vi "A-Lockin_Vsg.vi"(8 "error in (no error)":errorcluster, 9 "Channels: AO":T1={"AO amp (V)"=[0.0002, 0.0, 0.0, 0.0, 0.0, 0.0, 0.0, 0.0], "AO DC (V)"=[0.00025, 0.0, 0.0, 0.0, 0.0, 0.0, 0.0, 0.0], "AO f (Hz)"=[13.0, 13.0, 13.0, 13.0, 13.0, 13.0, 13.0, 13.0], "AO phi (deg)"=[0.0, 0.0, 0.0, 0.0, 0.0, 0.0, 0.0, 0.0], "function"=[enum."Sine Wave", enum."Sine Wave", enum."Sine Wave", enum."Sine Wave", enum."Sine Wave", enum."Sine Wave", enum."Sine Wave", enum."Sine Wave"]} {"AO f (Hz)" min=0.001 max=10000.0; "AO DC (V)" format="%#_6p"; "AO amp (V)" format="%#_6p"}, 10 "Comments":string="SA03036H\nsweep Vsg:-150m to 700m, 500u steps\nB 7T to -7T\nVbg =-3.9V\nT: 50mK\n\nlockin\n\nI+/-: 4/28 200uV ac+ 250u dc bias, 13Hz\nV1+/-: 3/27\nV2+/- 2/6\nV3+/V3-: 7/8\nVsg: 1\nVbg :26\n\ntc 300ms order 2", 11 "ITX folder":string="4L4Lockinfieldsweep") -> (0 "error out":errorcluster)   [LabVIEW 2016, in "Transport.lvclass"]
uses:
  Transport.lvclass
  <userlib>/LevyLab/Lockin-Multichannel/Typedefs/AO-cluster.ctl
  <userlib>/LevyLab/Lockin-Multichannel/Typedefs/AO_Amp-array.ctl
  <userlib>/LevyLab/Lockin-Multichannel/Typedefs/AO_DC-array.ctl
  <userlib>/LevyLab/Lockin-Multichannel/Typedefs/AO_f-array.ctl
  <userlib>/LevyLab/Lockin-Multichannel/Typedefs/AO_phi-array.ctl
  <userlib>/LevyLab/Lockin-Multichannel/Typedefs/Function-array.ctl
  <userlib>/LevyLab/Lockin-Multichannel/Typedefs/Function-enum.ctl
  SMOs/SweepControl/SweepControl.lvclass
  subVI/ITX_Global.vi
  <userlib>/LevyLab/Levylab Instruments/Instrument.lvclass
  <userlib>/LevyLab/LV to ITX/LVtoITX.lvclass
panel:
  in  "Tab Control":enum32{"lockin/SG Control", "Data"}(tab)
  in  "SweepControl.lvclass":refnum<class "SweepControl.lvclass">
  in  "Vmax (end)":dbl=0.7 format="%#_3p"
  in  "Vmin (start)":dbl=-0.15 format="%#_3p"
  in  "dV":dbl=0.0005 format="%#_3p"
  out "T (mK)":dbl
  in  "wait after setting Vsg (ms)":u32
  in  "Initial wait (ms)":u32=10000
  in  "side gate channel":i32=1
  in  "Physical Channel":tag="Dev2/ao0" caption="Back Gate Channel"
  in  "Sweep":enum16{"Vsg", "Vbg"}(ring)
  in  "cycles (1,2,...)":i32=1 min=1 step=1
  in  "phase":dbl
  out "ramp rate":dbl=0.2 format="%#_13g"
  out "Field":dbl=0.5 format="%#_13g"
  in  "function (ramp)":enum16{"Ramp", "Triangle", "Sine"}(ring)
  in  "set \"Vsg\" to initial value?":bool
  out "time (ms)":u32=76
  out "G 4T":cluster{"Y":dbl[], "Y":dbl[]}[](graph)
  out "Lockins":cluster{"Y":dbl[], "Y":dbl[]}[](graph)
  out "Lockins 2":cluster{"Y":dbl[], "Y":dbl[]}[](graph)
  # "0"
  # "1"
  # "2"
  # "3"
  # "4"
  # "5"
  # "6"
  # "7"
  # "dynamically name the traces"
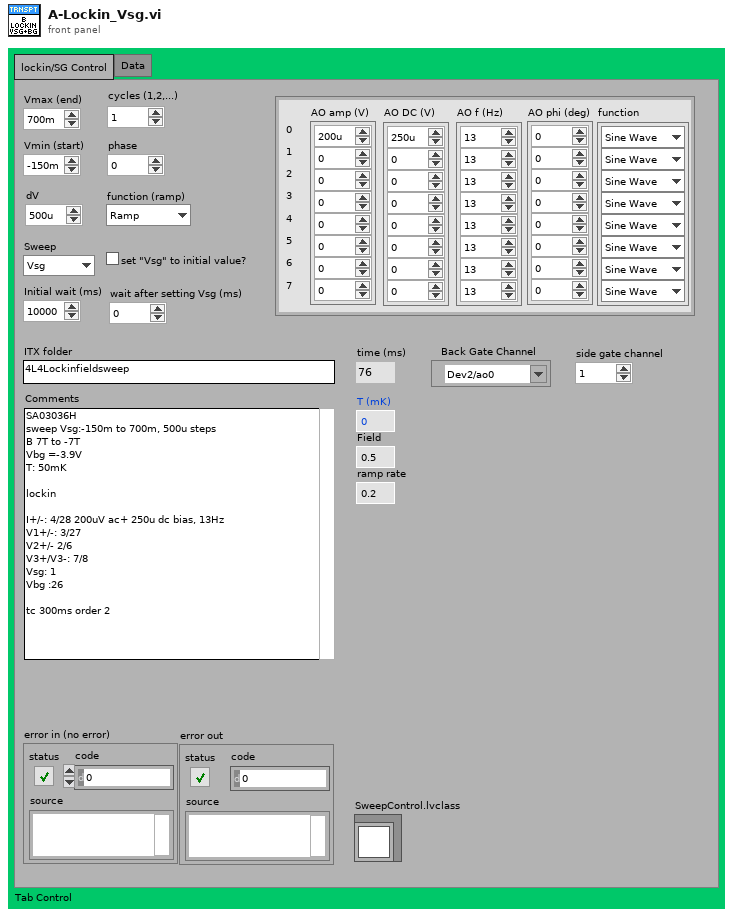
[diagram p1: front panel]
types:
  T1 = typedef "AO-cluster.ctl" = cluster{"AO amp (V)":T2, "AO DC (V)":T3, "AO f (Hz)":T4, "AO phi (deg)":T5, "function":T6}
  T2 = typedef "AO_Amp-array.ctl" = dbl[]
  T3 = typedef "AO_DC-array.ctl" = dbl[]
  T4 = typedef "AO_f-array.ctl" = dbl[]
  T5 = typedef "AO_phi-array.ctl" = dbl[]
  T6 = typedef "Function-array.ctl" = T7[]
  T7 = typedef "Function-enum.ctl" = enum16{"Sine Wave", "Triangle Wave", "Square Wave", "Sawtooth Wave"}
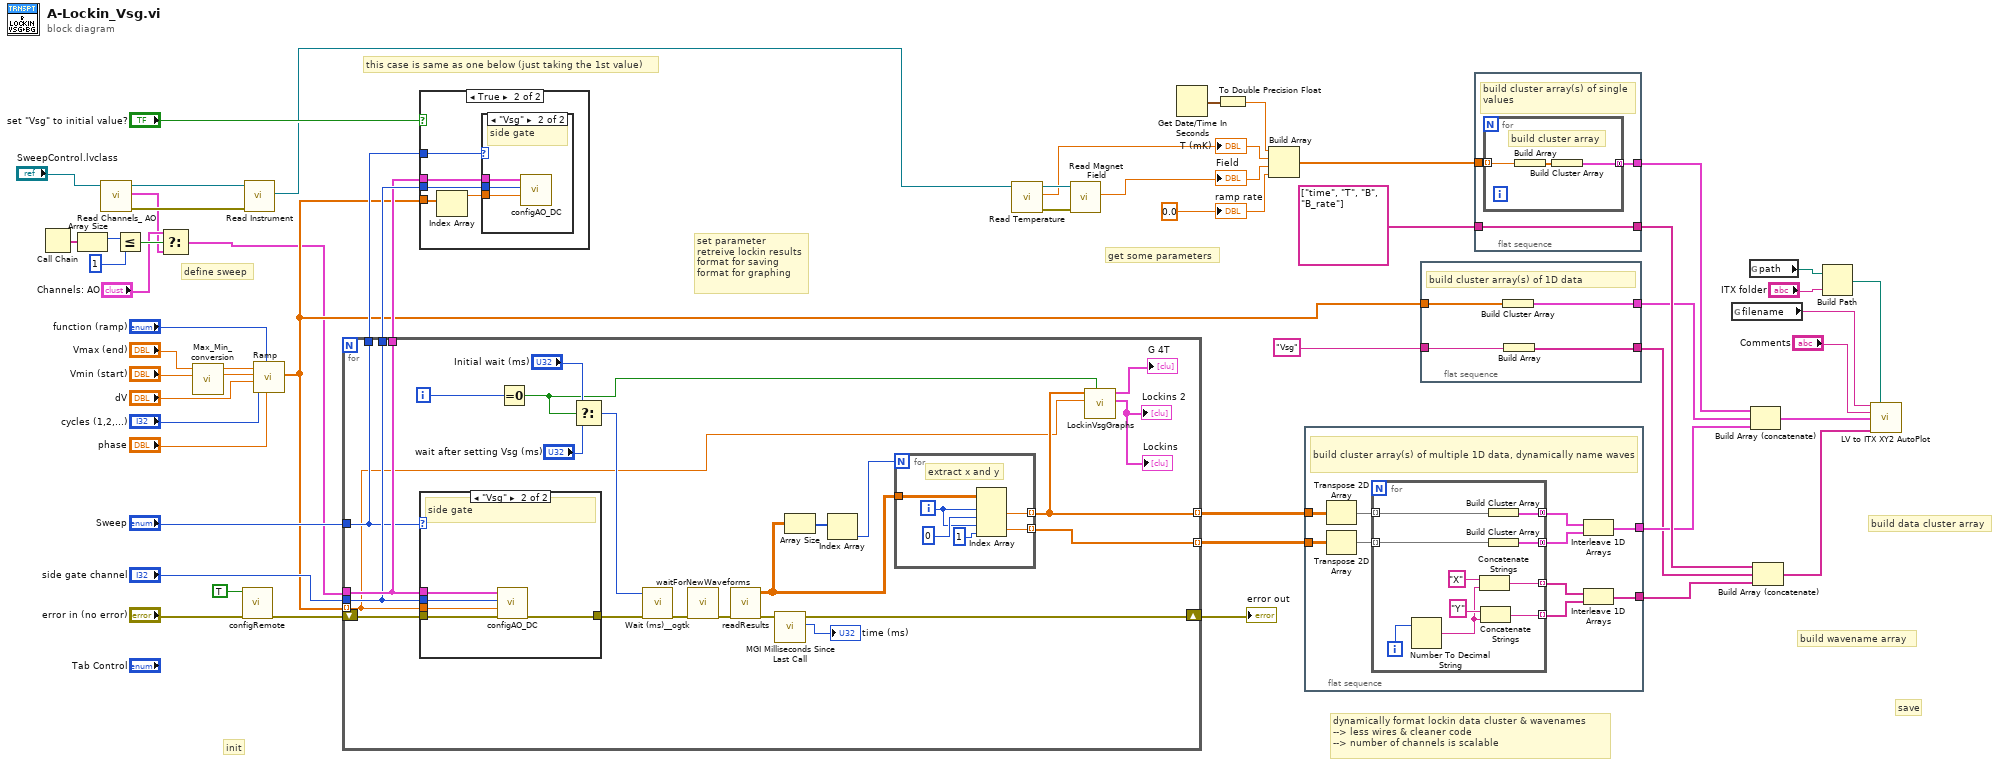
[diagram p0: block diagram]
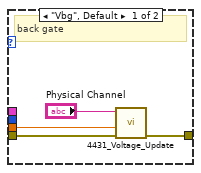
[diagram p2: hidden frame]
diagram:
  w19 = 0.0
  # "define sweep"
  # "get some parameters"
  # "set parameter\nretreive lockin results\nformat for saving\nformat for graphing"
  # "save"
  # "this case is same as one below (just taking the 1st value)"
  # "init"
  # "build data cluster array"
  # "build wavename array"
  # "dynamically format lockin data cluster & wavenames\n--> less wires & cleaner code\n--> number of channels is scalable"
  n1 = Call Chain() -> (call chain=w7:string[])
  n2 = Array Size(array=w7) -> (size(s)=w6:i32)
  n3 = call-dynamic "Read Channels_ AO.vi"("SweepControl in"="SweepControl.lvclass") -> ("error out"=w14:errorcluster, "Channels: AO"=w2:T1, "SweepControl out"=w13:refnum<class "SweepControl.lvclass">)  [unwired: 8 in]
  n4 = Less Or Equal?(x=w6, y=1) -> (x <= y?=w4:bool)
  n5 = Select(t="Channels: AO", s=w4, f=w2) -> (s? t:f=w1:T1)
  n6 = call <userlib>:"Max_Min_conversion.vi"("Min"="Vmin (start)", "Max"="Vmax (end)") -> ("offset"=w52:dbl, "Amplitude"=w53:dbl)  [unwired: 8 in]
  n7 = call <userlib>:"configRemote.vi"("error in (no error)"="error in (no error)", "Remote Mode"=TRUE) -> ("error out"=w43:errorcluster)  [unwired: 9 in]
  n8 = call-dynamic "Read Instrument.vi"("error in (no error)"=w14, "SweepControl in"=w13) -> ("Instrument.lvclass"=w12:refnum<class "Instrument.lvclass">)  [unwired: 7 in, 2 out]
  n9 = call <userlib>:"Ramp.vi"("phase"="phase", "function (ramp)"="function (ramp)", "cycles (1,2,...)"="cycles (1,2,...)", "step size"="dV", "offset"=w52, "amplitude"=w53) -> ("Waveform Graph"=w16:dbl[])  [unwired: 3 in, 2 out]
  n10 = for {
    tunnel: w1 -> [w78]
    tunnel: w16 -> [w56] mode=indexing
    tunnel: "Sweep" -> [w76]
    tunnel: "side gate channel" -> [w77]
    tunnel: [w78] -> w42
    tunnel: [w77] -> w46
    tunnel: [w76] -> w45
    shift-right: [w72] -> w34
    shift-left: w43 -> [w75]
    tunnel: [w60] -> w37 mode=indexing
    tunnel: [w62] -> w36 mode=indexing
    i -> [w73]
    n11 = case shown="\"Vsg\"" w76 {
      tunnel: w78 -> [_ w93]
      tunnel: w56 -> [w88 w91]
      tunnel: w77 -> [_ w92]
      tunnel: w75 -> [w86 w90]
      tunnel: [w85 w89] -> w74
      frame "Vbg", Default {
        # "back gate"
        n12 = call "4431_Voltage_Update.vi"("error in"=w86, "Amplified output"=w88, "Physical Channel(s)"="Physical Channel") -> ("error out"=w85:errorcluster)  [unwired: 8 in]
      }
      frame "Vsg" {
        # "side gate"
        n13 = call <userlib>:"configAO_DC.vi"("error in (no error)"=w90, "new DC (V)"=w91, "AO Channel"=w92, "Channels: AO"=w93) -> ("error out"=w89:errorcluster)  [unwired: 6 in, 1 out]
      }
    }
    n14 = Equal To 0?(x=w73) -> (x = 0?=w59:bool)
    n15 = Select(t="Initial wait (ms)", s=w59, f="wait after setting Vsg (ms)") -> (s? t:f=w64:u32)
    n16 = call <userlib>:"Wait (ms)__ogtk.vi"("error in (no error)"=w74, "milliseconds to wait"=w64) -> ("error out"=w67:errorcluster)  [unwired: 8 in, 1 out]
    n17 = call <userlib>:"waitForNewWaveforms.vi"("error in (no error)"=w67) -> ("error out"=w61:errorcluster)  [unwired: 9 in, 1 out]
    n18 = call <userlib>:"readResults.vi"("error in (no error)"=w61) -> ("error out"=w71:errorcluster, "Results"=w70:dbl[][])  [unwired: 8 in, 1 out]
    n19 = call <userlib>:"MGI Milliseconds Since Last Call.vi"("Error In"=w71) -> ("ms"=→"time (ms)":u32, "Error Out"=w72:errorcluster)  [unwired: 5 in]
    n20 = Array Size(array=w70) -> (size(s)=w69:i32[])
    n21 = Index Array(array=w69) -> (element=w68:i32)  [unwired: 1 in]
    n22 = for {
      N: w68 -> [_]
      tunnel: w70 -> [w82]
      tunnel: [w80] -> w60 mode=indexing
      tunnel: [w79] -> w62 mode=indexing
      i -> [w81]
      # "extract x and y"
      n23 = Index Array(array=w82, index (row) #1=w81, index (col) #1=0 ("disabled index (col)"), index (row) #2=w81, index (col) #2=1 ("disabled index (col)")) -> (element #1=w80:dbl, element #2=w79:dbl)
    }
    n24 = call "LockinVsgGraphs.vi"("reset?"=w59, "X in"=w56, "Y array in"=w60) -> ("Y vs X"=→"Lockins" →"Lockins 2":cluster{"Y":dbl[], "Y":dbl[]}[], "Array out"=→"G 4T":cluster{"Y":dbl[], "Y":dbl[]}[])  [unwired: 7 in]
  }
  "error out" <- w34
  n25 = case shown="True" "set \"Vsg\" to initial value?" {
    tunnel: w42 -> [_ w98]
    tunnel: w16 -> [_ w97]
    tunnel: w46 -> [_ w95]
    tunnel: w45 -> [_ w96]
    frame False {
    }
    frame True {
      n26 = Index Array(array=w97) -> (element=w94:dbl)  [unwired: 1 in]
      n27 = case shown="\"Vsg\"" w96 {
        tunnel: w98 -> [_ w99]
        tunnel: w94 -> [_ w100]
        tunnel: w95 -> [_ w101]
        frame "Vbg", Default {
          # "back gate"
        }
        frame "Vsg" {
          # "side gate"
          n28 = call <userlib>:"configAO_DC.vi"("new DC (V)"=w100, "AO Channel"=w101, "Channels: AO"=w99) -> ()  [unwired: 7 in, 2 out]
        }
      }
    }
  }
  n29 = call-dynamic "Read Temperature.vi"("Instrument in"=w12) -> ("error out"=w8:errorcluster, "Temperature (K)"=w10:dbl, "Instrument out"=w11:refnum<class "Instrument.lvclass">)  [unwired: 7 in, 1 out]
  "T (mK)" <- w10
  n30 = call-dynamic "Read Magnet Field.vi"("error in (no error)"=w8, "Instrument in"=w11) -> ("Field (T)"=w9:dbl)  [unwired: 6 in, 3 out]
  "Field" <- w9
  n31 = Get Date/Time In Seconds() -> (seconds since 1Jan1904=w22:timestamp)
  n32 = To Double Precision Float(number=w22) -> (double precision float=w20:dbl)
  n33 = Build Array(w20, w10, w9, w19) -> (w21:dbl[])
  n34 = flat-sequence {
    tunnel: w37 -> [w111]
    tunnel: w36 -> [w110]
    tunnel: [w103] -> w30
    tunnel: [w102] -> w27
    frame #0 {
      # "build cluster array(s) of multiple 1D data, dynamically name waves"
      n35 = Transpose 2D Array(2D array=w111) -> (transposed array=w109:dbl[][])
      n36 = Transpose 2D Array(2D array=w110) -> (transposed array=w108:dbl[][])
      n37 = for {
        tunnel: w109 -> [w121] mode=indexing
        tunnel: w108 -> [w120] mode=indexing
        tunnel: [w119] -> w107 mode=concatenating
        tunnel: [w118] -> w106 mode=concatenating
        tunnel: [w113] -> w105 mode=indexing
        tunnel: [w112] -> w104 mode=indexing
        i -> [w115]
        n38 = Number To Decimal String(number=w115) -> (decimal integer string=w114:string)  [unwired: 1 in]
        n39 = Concatenate Strings("X" ("wavenames"), w114) -> (w113:string)
        n40 = Concatenate Strings("Y" ("wavenames"), w114) -> (w112:string)
        n41 = Build Cluster Array(w121) -> (w119:cluster{dbl[]}[])
        n42 = Build Cluster Array(w120) -> (w118:cluster{dbl[]}[])
      }
      n43 = Interleave 1D Arrays(w107, w106) -> (w102:cluster{dbl[]}[])
      n44 = Interleave 1D Arrays(w105, w104) -> (w103:string[])
    }
  }
  n45 = flat-sequence {
    tunnel: [w122] -> w26
    tunnel: w16 -> [w125]
    tunnel: [w124] -> w25
    tunnel: "Vsg" ("wavenames") -> [w123]
    frame #0 {
      # "build cluster array(s) of 1D data"
      n46 = Build Cluster Array(w125) -> (w124:cluster{"Waveform Graph":dbl[]}[])
      n47 = Build Array(w123) -> (w122:string[])
    }
  }
  n48 = flat-sequence {
    tunnel: [w128] -> w33
    tunnel: [w126] -> w31
    tunnel: w21 -> [w127]
    tunnel: string[] ["time", "T", "B", "B_rate"] ("wavenames (.Vx, etc)") -> [w126]
    frame #0 {
      # "build cluster array(s) of single values"
      n49 = for {
        tunnel: [w130] -> w128 mode=concatenating
        tunnel: w127 -> [w129] mode=indexing
        # "build cluster array"
        n50 = Build Array(w129) -> (w131:dbl[])
        n51 = Build Cluster Array(w131) -> (w130:cluster{dbl[]}[])
      }
    }
  }
  n52 = global read "ITX_Global.vi" "filename"() -> (w39:string)
  n53 = global read "ITX_Global.vi" "path"() -> (w24:path)
  n54 = Build Array (concatenate)(w33, w25, w27) -> (w32:cluster{"Waveform Graph":dbl[]}[])
  n55 = Build Array (concatenate)(w31, w26, w30) -> (w35:string[])
  n56 = Build Path(base path=w24, name or relative path="ITX folder") -> (appended path=w55:path)
  n57 = call <userlib>:"LV to ITX XY2 AutoPlot.vi"("filename"=w39, "path"=w55, "Notes"="Comments", "Data"=w32, "wavenames (.Vx, etc)"=w35) -> ()  [unwired: 10 in, 1 out]
  "ramp rate" <- w19
